vi "IR Stimulus DLL (SubVI).vi"(5 "GALVO Calibration Data":T1, 7 "Cycle Time (ms)":i32=50, 8 "LASER Intensity (%)":dbl format="%#_13g", 11 "irData":i32[](array[numeric])) -> (0 "Max. LASER Power (W)":dbl, 3 "daqData":dbl[][](array[numeric]))   [LabVIEW 2020]
uses:
  Controls (HOST)/IR GALVO Cal Data.ctl
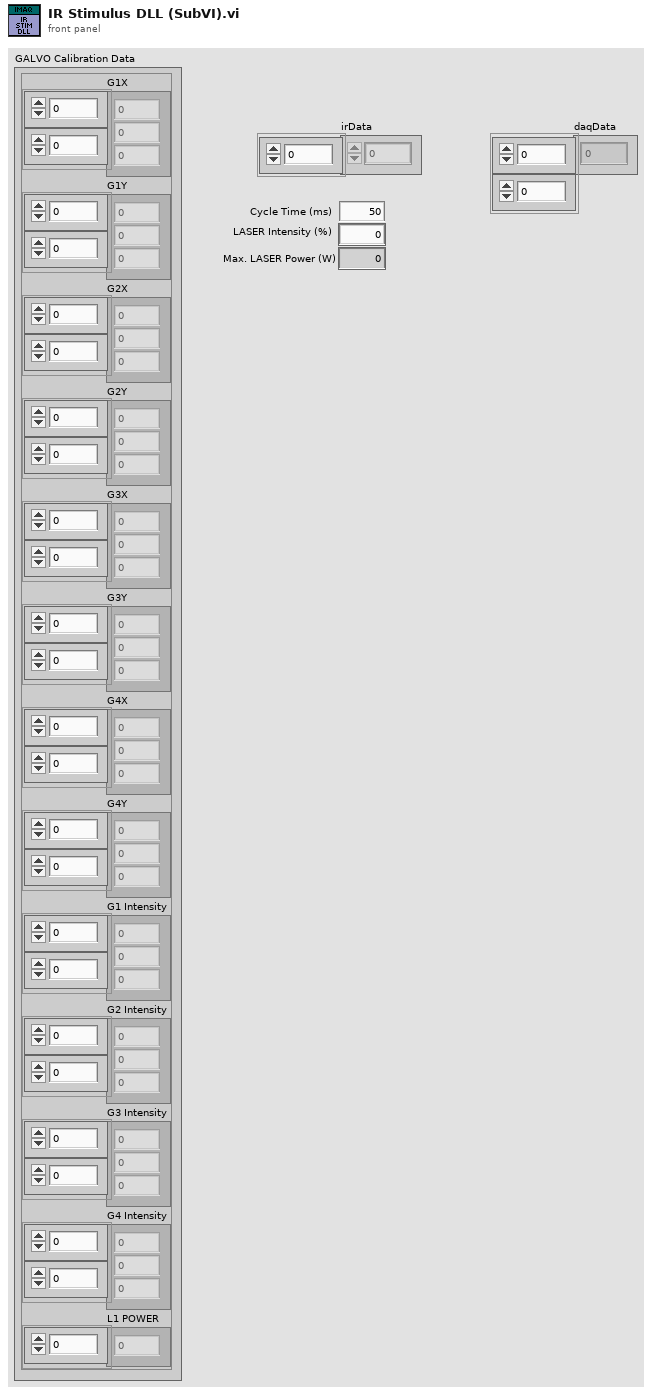
[diagram p1: front panel]
types:
  T1 = typedef "IR GALVO Cal Data.ctl" = cluster{"G1X":dbl[][], "G1Y":dbl[][], "G2X":dbl[][], "G2Y":dbl[][], "G3X":dbl[][], "G3Y":dbl[][], "G4X":dbl[][], "G4Y":dbl[][], "G1 Intensity":dbl[][], "G2 Intensity":dbl[][], "G3 Intensity":dbl[][], "G4 Intensity":dbl[][], "L1 POWER":dbl[]}
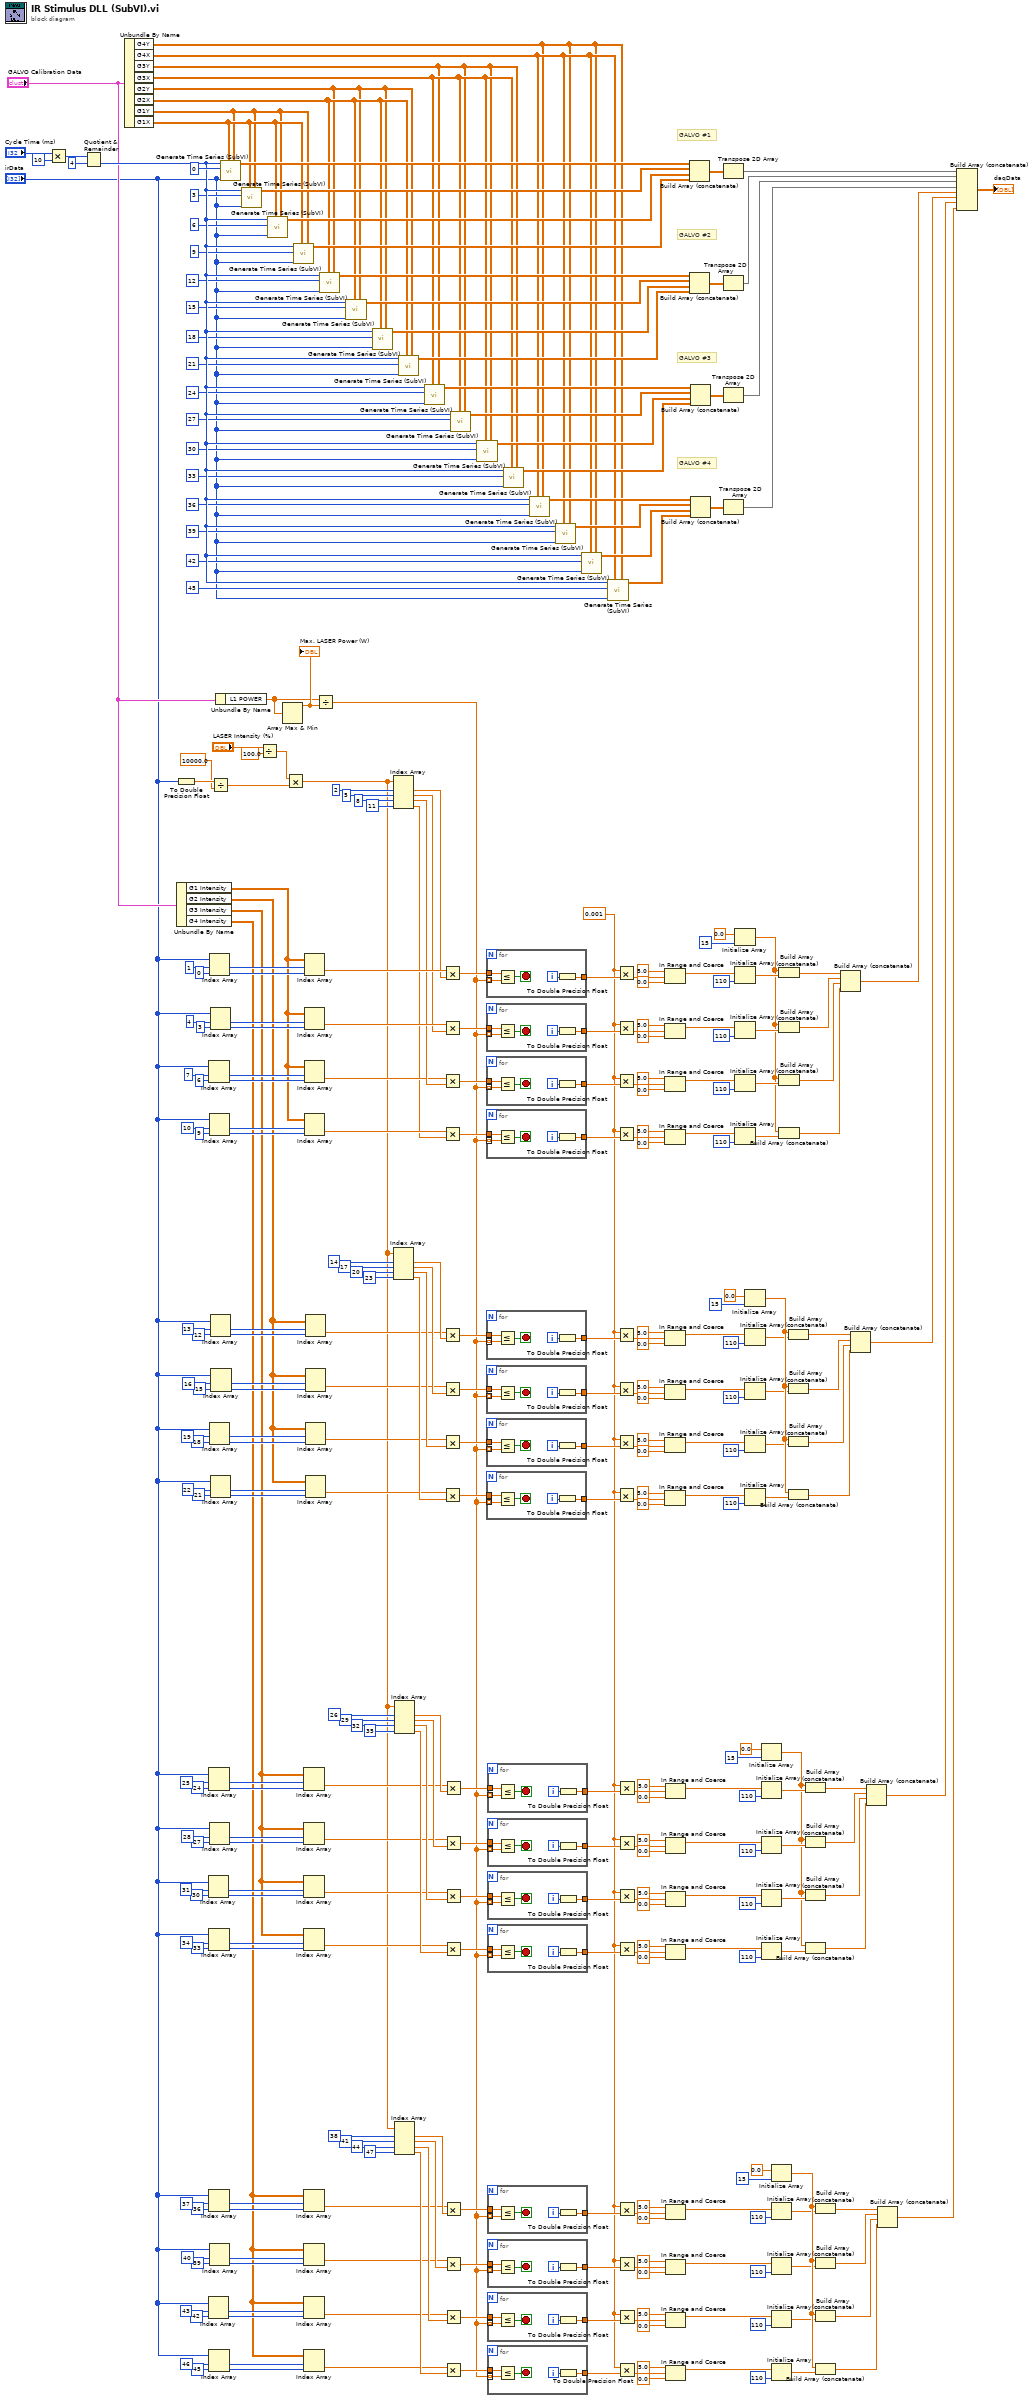
[diagram p0: block diagram]
diagram:
  w68 = 0.001 ("x")
  # "GALVO #4"
  # "GALVO #3"
  # "GALVO #2"
  # "GALVO #1"
  n1 = Multiply(x="Cycle Time (ms)", y=10) -> (x*y=w341:i32)
  n2 = Quotient & Remainder(x=w341, y=4) -> (floor(x/y)=w338:i32)  [unwired: 1 out]
  n3 = Unbundle By Name("GALVO Calibration Data") -> ("G4Y"=w290:dbl[][], "G4X"=w291:dbl[][], "G3Y"=w292:dbl[][], "G3X"=w293:dbl[][], "G2Y"=w294:dbl[][], "G2X"=w295:dbl[][], "G1Y"=w296:dbl[][], "G1X"=w297:dbl[][])
  n4 = To Double Precision Float(number="irData") -> (double precision float=w209:dbl[])
  n5 = Unbundle By Name("GALVO Calibration Data") -> ("G1 Intensity"=w256:dbl[][], "G2 Intensity"=w239:dbl[][], "G3 Intensity"=w238:dbl[][], "G4 Intensity"=w221:dbl[][])
  n6 = Index Array(array="irData", index #1=31 ("index"), index #2=30 ("index")) -> (element #1=w241:i32, element #2=w242:i32)
  n7 = Index Array(array="irData", index #1=43 ("index"), index #2=42 ("index")) -> (element #1=w236:i32, element #2=w235:i32)
  n8 = Index Array(array="irData", index #1=7 ("index"), index #2=6 ("index")) -> (element #1=w275:i32, element #2=w276:i32)
  n9 = Index Array(array="irData", index #1=25 ("index"), index #2=24 ("index")) -> (element #1=w254:i32, element #2=w253:i32)
  n10 = Index Array(array="irData", index #1=34 ("index"), index #2=33 ("index")) -> (element #1=w246:i32, element #2=w245:i32)
  n11 = Index Array(array="irData", index #1=37 ("index"), index #2=36 ("index")) -> (element #1=w223:i32, element #2=w224:i32)
  n12 = Index Array(array="irData", index #1=46 ("index"), index #2=45 ("index")) -> (element #1=w231:i32, element #2=w232:i32)
  n13 = Index Array(array="irData", index #1=1 ("index"), index #2=0 ("index")) -> (element #1=w288:i32, element #2=w287:i32)
  n14 = Index Array(array="irData", index #1=10 ("index"), index #2=9 ("index")) -> (element #1=w280:i32, element #2=w279:i32)
  n15 = Index Array(array="irData", index #1=19 ("index"), index #2=18 ("index")) -> (element #1=w271:i32, element #2=w270:i32)
  n16 = Index Array(array="irData", index #1=28 ("index"), index #2=27 ("index")) -> (element #1=w249:i32, element #2=w250:i32)
  n17 = Index Array(array="irData", index #1=40 ("index"), index #2=39 ("index")) -> (element #1=w228:i32, element #2=w227:i32)
  n18 = Index Array(array="irData", index #1=4 ("index"), index #2=3 ("index")) -> (element #1=w283:i32, element #2=w284:i32)
  n19 = Index Array(array="irData", index #1=13 ("index"), index #2=12 ("index")) -> (element #1=w258:i32, element #2=w259:i32)
  n20 = Index Array(array="irData", index #1=22 ("index"), index #2=21 ("index")) -> (element #1=w266:i32, element #2=w267:i32)
  n21 = Divide(x=w209, y=10000.0 ("LASER Intensity (%)")) -> (x/y=w208:dbl[])
  n22 = Index Array(array="irData", index #1=16 ("index"), index #2=15 ("index")) -> (element #1=w263:i32, element #2=w262:i32)
  n23 = Unbundle By Name("GALVO Calibration Data") -> ("L1 POWER"=w216:dbl[])
  n24 = call "Generate Time Series (SubVI).vi"("GY"=w296, "GX"=w297, "irData"="irData", "Start Index"=0, "N Steps"=w338) -> ("daqData"=w322:dbl[][])  [unwired: 6 in]
  n25 = call "Generate Time Series (SubVI).vi"("GY"=w296, "GX"=w297, "irData"="irData", "Start Index"=3, "N Steps"=w338) -> ("daqData"=w321:dbl[][])  [unwired: 6 in]
  n26 = Divide(x="LASER Intensity (%)", y=100.0 ("x")) -> (x/y=w86:dbl)
  n27 = call "Generate Time Series (SubVI).vi"("GY"=w296, "GX"=w297, "irData"="irData", "Start Index"=6, "N Steps"=w338) -> ("daqData"=w320:dbl[][])  [unwired: 6 in]
  n28 = Array Max & Min(array=w216) -> (max value=w217:dbl)  [unwired: 3 out]
  "Max. LASER Power (W)" <- w217
  n29 = Multiply(x=w86, y=w208) -> (x*y=w92:dbl[])
  n30 = call "Generate Time Series (SubVI).vi"("GY"=w296, "GX"=w297, "irData"="irData", "Start Index"=9, "N Steps"=w338) -> ("daqData"=w319:dbl[][])  [unwired: 6 in]
  n31 = Index Array(array=w238, index (row)=w254, index (col)=w253) -> (element=w120:dbl)
  n32 = Index Array(array=w238, index (row)=w249, index (col)=w250) -> (element=w119:dbl)
  n33 = Index Array(array=w238, index (row)=w241, index (col)=w242) -> (element=w118:dbl)
  n34 = Index Array(array=w238, index (row)=w246, index (col)=w245) -> (element=w117:dbl)
  n35 = Index Array(array=w221, index (row)=w223, index (col)=w224) -> (element=w90:dbl)
  n36 = Index Array(array=w221, index (row)=w228, index (col)=w227) -> (element=w89:dbl)
  n37 = Index Array(array=w221, index (row)=w236, index (col)=w235) -> (element=w88:dbl)
  n38 = Index Array(array=w221, index (row)=w231, index (col)=w232) -> (element=w87:dbl)
  n39 = Index Array(array=w256, index (row)=w288, index (col)=w287) -> (element=w201:dbl)
  n40 = Index Array(array=w256, index (row)=w283, index (col)=w284) -> (element=w194:dbl)
  n41 = Index Array(array=w256, index (row)=w275, index (col)=w276) -> (element=w183:dbl)
  n42 = Index Array(array=w256, index (row)=w280, index (col)=w279) -> (element=w176:dbl)
  n43 = Index Array(array=w239, index (row)=w258, index (col)=w259) -> (element=w148:dbl)
  n44 = Index Array(array=w239, index (row)=w263, index (col)=w262) -> (element=w147:dbl)
  n45 = Index Array(array=w239, index (row)=w271, index (col)=w270) -> (element=w146:dbl)
  n46 = Index Array(array=w239, index (row)=w266, index (col)=w267) -> (element=w145:dbl)
  n47 = Divide(x=w216, y=w217) -> (x/y=w91:dbl[])
  n48 = call "Generate Time Series (SubVI).vi"("GY"=w294, "GX"=w295, "irData"="irData", "Start Index"=12, "N Steps"=w338) -> ("daqData"=w318:dbl[][])  [unwired: 6 in]
  n49 = call "Generate Time Series (SubVI).vi"("GY"=w294, "GX"=w295, "irData"="irData", "Start Index"=15, "N Steps"=w338) -> ("daqData"=w317:dbl[][])  [unwired: 6 in]
  n50 = call "Generate Time Series (SubVI).vi"("GY"=w294, "GX"=w295, "irData"="irData", "Start Index"=18, "N Steps"=w338) -> ("daqData"=w316:dbl[][])  [unwired: 6 in]
  n51 = Index Array(array=w92, index #1=2 ("index"), index #2=5 ("index"), index #3=8 ("index"), index #4=11 ("index")) -> (element #1=w193:dbl, element #2=w185:dbl, element #3=w184:dbl, element #4=w175:dbl)
  n52 = Index Array(array=w92, index #1=14 ("index"), index #2=17 ("index"), index #3=20 ("index"), index #4=23 ("index")) -> (element #1=w161:dbl, element #2=w166:dbl, element #3=w167:dbl, element #4=w172:dbl)
  n53 = Index Array(array=w92, index #1=26 ("index"), index #2=29 ("index"), index #3=32 ("index"), index #4=35 ("index")) -> (element #1=w132:dbl, element #2=w127:dbl, element #3=w126:dbl, element #4=w121:dbl)
  n54 = Index Array(array=w92, index #1=38 ("index"), index #2=41 ("index"), index #3=44 ("index"), index #4=47 ("index")) -> (element #1=w105:dbl, element #2=w110:dbl, element #3=w111:dbl, element #4=w116:dbl)
  n55 = call "Generate Time Series (SubVI).vi"("GY"=w294, "GX"=w295, "irData"="irData", "Start Index"=21, "N Steps"=w338) -> ("daqData"=w315:dbl[][])  [unwired: 6 in]
  n56 = call "Generate Time Series (SubVI).vi"("GY"=w292, "GX"=w293, "irData"="irData", "Start Index"=24, "N Steps"=w338) -> ("daqData"=w314:dbl[][])  [unwired: 6 in]
  n57 = Multiply(x=w201, y=w193) -> (x*y=w202:dbl)
  n58 = Multiply(x=w194, y=w185) -> (x*y=w200:dbl)
  n59 = Multiply(x=w183, y=w184) -> (x*y=w186:dbl)
  n60 = Multiply(x=w176, y=w175) -> (x*y=w182:dbl)
  n61 = Multiply(x=w148, y=w161) -> (x*y=w156:dbl)
  n62 = Multiply(x=w147, y=w166) -> (x*y=w157:dbl)
  n63 = Multiply(x=w146, y=w167) -> (x*y=w165:dbl)
  n64 = Multiply(x=w145, y=w172) -> (x*y=w168:dbl)
  n65 = Multiply(x=w120, y=w132) -> (x*y=w137:dbl)
  n66 = Multiply(x=w119, y=w127) -> (x*y=w136:dbl)
  n67 = Multiply(x=w118, y=w126) -> (x*y=w128:dbl)
  n68 = Multiply(x=w117, y=w121) -> (x*y=w125:dbl)
  n69 = Multiply(x=w90, y=w105) -> (x*y=w100:dbl)
  n70 = Multiply(x=w89, y=w110) -> (x*y=w101:dbl)
  n71 = Multiply(x=w88, y=w111) -> (x*y=w109:dbl)
  n72 = Multiply(x=w87, y=w116) -> (x*y=w112:dbl)
  n73 = call "Generate Time Series (SubVI).vi"("GY"=w292, "GX"=w293, "irData"="irData", "Start Index"=27, "N Steps"=w338) -> ("daqData"=w313:dbl[][])  [unwired: 6 in]
  n74 = call "Generate Time Series (SubVI).vi"("GY"=w292, "GX"=w293, "irData"="irData", "Start Index"=30, "N Steps"=w338) -> ("daqData"=w312:dbl[][])  [unwired: 6 in]
  n75 = for {
    tunnel: w91 -> [w348] mode=indexing
    tunnel: [w345] -> w215
    tunnel: w202 -> [w344]
    i -> [w346]
    stop <- w347 stop-if-true
    n76 = Less Or Equal?(x=w344, y=w348) -> (x <= y?=w347:bool)
    n77 = To Double Precision Float(number=w346) -> (double precision float=w345:dbl)
  }
  n78 = for {
    tunnel: w91 -> [w353] mode=indexing
    tunnel: [w350] -> w197
    tunnel: w200 -> [w349]
    i -> [w351]
    stop <- w352 stop-if-true
    n79 = Less Or Equal?(x=w349, y=w353) -> (x <= y?=w352:bool)
    n80 = To Double Precision Float(number=w351) -> (double precision float=w350:dbl)
  }
  n81 = for {
    tunnel: w91 -> [w358] mode=indexing
    tunnel: [w355] -> w189
    tunnel: w186 -> [w354]
    i -> [w356]
    stop <- w357 stop-if-true
    n82 = Less Or Equal?(x=w354, y=w358) -> (x <= y?=w357:bool)
    n83 = To Double Precision Float(number=w356) -> (double precision float=w355:dbl)
  }
  n84 = for {
    tunnel: w91 -> [w363] mode=indexing
    tunnel: [w360] -> w179
    tunnel: w182 -> [w359]
    i -> [w361]
    stop <- w362 stop-if-true
    n85 = Less Or Equal?(x=w359, y=w363) -> (x <= y?=w362:bool)
    n86 = To Double Precision Float(number=w361) -> (double precision float=w360:dbl)
  }
  n87 = for {
    tunnel: w91 -> [w368] mode=indexing
    tunnel: [w365] -> w151
    tunnel: w156 -> [w364]
    i -> [w366]
    stop <- w367 stop-if-true
    n88 = Less Or Equal?(x=w364, y=w368) -> (x <= y?=w367:bool)
    n89 = To Double Precision Float(number=w366) -> (double precision float=w365:dbl)
  }
  n90 = for {
    tunnel: w91 -> [w373] mode=indexing
    tunnel: [w370] -> w158
    tunnel: w157 -> [w369]
    i -> [w371]
    stop <- w372 stop-if-true
    n91 = Less Or Equal?(x=w369, y=w373) -> (x <= y?=w372:bool)
    n92 = To Double Precision Float(number=w371) -> (double precision float=w370:dbl)
  }
  n93 = for {
    tunnel: w91 -> [w378] mode=indexing
    tunnel: [w375] -> w164
    tunnel: w165 -> [w374]
    i -> [w376]
    stop <- w377 stop-if-true
    n94 = Less Or Equal?(x=w374, y=w378) -> (x <= y?=w377:bool)
    n95 = To Double Precision Float(number=w376) -> (double precision float=w375:dbl)
  }
  n96 = for {
    tunnel: w91 -> [w383] mode=indexing
    tunnel: [w380] -> w169
    tunnel: w168 -> [w379]
    i -> [w381]
    stop <- w382 stop-if-true
    n97 = Less Or Equal?(x=w379, y=w383) -> (x <= y?=w382:bool)
    n98 = To Double Precision Float(number=w381) -> (double precision float=w380:dbl)
  }
  n99 = for {
    tunnel: w91 -> [w388] mode=indexing
    tunnel: [w385] -> w142
    tunnel: w137 -> [w384]
    i -> [w386]
    stop <- w387 stop-if-true
    n100 = Less Or Equal?(x=w384, y=w388) -> (x <= y?=w387:bool)
    n101 = To Double Precision Float(number=w386) -> (double precision float=w385:dbl)
  }
  n102 = for {
    tunnel: w91 -> [w393] mode=indexing
    tunnel: [w390] -> w135
    tunnel: w136 -> [w389]
    i -> [w391]
    stop <- w392 stop-if-true
    n103 = Less Or Equal?(x=w389, y=w393) -> (x <= y?=w392:bool)
    n104 = To Double Precision Float(number=w391) -> (double precision float=w390:dbl)
  }
  n105 = for {
    tunnel: w91 -> [w398] mode=indexing
    tunnel: [w395] -> w129
    tunnel: w128 -> [w394]
    i -> [w396]
    stop <- w397 stop-if-true
    n106 = Less Or Equal?(x=w394, y=w398) -> (x <= y?=w397:bool)
    n107 = To Double Precision Float(number=w396) -> (double precision float=w395:dbl)
  }
  n108 = for {
    tunnel: w91 -> [w403] mode=indexing
    tunnel: [w400] -> w124
    tunnel: w125 -> [w399]
    i -> [w401]
    stop <- w402 stop-if-true
    n109 = Less Or Equal?(x=w399, y=w403) -> (x <= y?=w402:bool)
    n110 = To Double Precision Float(number=w401) -> (double precision float=w400:dbl)
  }
  n111 = for {
    tunnel: w91 -> [w408] mode=indexing
    tunnel: [w405] -> w95
    tunnel: w100 -> [w404]
    i -> [w406]
    stop <- w407 stop-if-true
    n112 = Less Or Equal?(x=w404, y=w408) -> (x <= y?=w407:bool)
    n113 = To Double Precision Float(number=w406) -> (double precision float=w405:dbl)
  }
  n114 = for {
    tunnel: w91 -> [w413] mode=indexing
    tunnel: [w410] -> w102
    tunnel: w101 -> [w409]
    i -> [w411]
    stop <- w412 stop-if-true
    n115 = Less Or Equal?(x=w409, y=w413) -> (x <= y?=w412:bool)
    n116 = To Double Precision Float(number=w411) -> (double precision float=w410:dbl)
  }
  n117 = for {
    tunnel: w91 -> [w418] mode=indexing
    tunnel: [w415] -> w108
    tunnel: w109 -> [w414]
    i -> [w416]
    stop <- w417 stop-if-true
    n118 = Less Or Equal?(x=w414, y=w418) -> (x <= y?=w417:bool)
    n119 = To Double Precision Float(number=w416) -> (double precision float=w415:dbl)
  }
  n120 = for {
    tunnel: w91 -> [w423] mode=indexing
    tunnel: [w420] -> w113
    tunnel: w112 -> [w419]
    i -> [w421]
    stop <- w422 stop-if-true
    n121 = Less Or Equal?(x=w419, y=w423) -> (x <= y?=w422:bool)
    n122 = To Double Precision Float(number=w421) -> (double precision float=w420:dbl)
  }
  n123 = call "Generate Time Series (SubVI).vi"("GY"=w292, "GX"=w293, "irData"="irData", "Start Index"=33, "N Steps"=w338) -> ("daqData"=w311:dbl[][])  [unwired: 6 in]
  n124 = call "Generate Time Series (SubVI).vi"("GY"=w290, "GX"=w291, "irData"="irData", "Start Index"=36, "N Steps"=w338) -> ("daqData"=w310:dbl[][])  [unwired: 6 in]
  n125 = call "Generate Time Series (SubVI).vi"("GY"=w290, "GX"=w291, "irData"="irData", "Start Index"=39, "N Steps"=w338) -> ("daqData"=w309:dbl[][])  [unwired: 6 in]
  n126 = call "Generate Time Series (SubVI).vi"("GY"=w290, "GX"=w291, "irData"="irData", "Start Index"=42, "N Steps"=w338) -> ("daqData"=w308:dbl[][])  [unwired: 6 in]
  n127 = call "Generate Time Series (SubVI).vi"("GY"=w290, "GX"=w291, "irData"="irData", "Start Index"=45, "N Steps"=w338) -> ("daqData"=w307:dbl[][])  [unwired: 6 in]
  n128 = Multiply(x=w68, y=w215) -> (x*y=w84:dbl)
  n129 = Multiply(x=w68, y=w197) -> (x*y=w83:dbl)
  n130 = Multiply(x=w68, y=w189) -> (x*y=w82:dbl)
  n131 = Multiply(x=w68, y=w179) -> (x*y=w81:dbl)
  n132 = Multiply(x=w68, y=w151) -> (x*y=w80:dbl)
  n133 = Multiply(x=w68, y=w158) -> (x*y=w79:dbl)
  n134 = Multiply(x=w68, y=w164) -> (x*y=w78:dbl)
  n135 = Multiply(x=w68, y=w169) -> (x*y=w77:dbl)
  n136 = Multiply(x=w68, y=w142) -> (x*y=w76:dbl)
  n137 = Multiply(x=w68, y=w135) -> (x*y=w75:dbl)
  n138 = Multiply(x=w68, y=w129) -> (x*y=w74:dbl)
  n139 = Multiply(x=w68, y=w124) -> (x*y=w73:dbl)
  n140 = Multiply(x=w68, y=w95) -> (x*y=w72:dbl)
  n141 = Multiply(x=w68, y=w102) -> (x*y=w71:dbl)
  n142 = Multiply(x=w68, y=w108) -> (x*y=w70:dbl)
  n143 = Multiply(x=w68, y=w113) -> (x*y=w69:dbl)
  n144 = In Range and Coerce(upper limit=5.0, x=w84, lower limit=0.0) -> (coerced(x)=w205:dbl)  [unwired: 1 out]
  n145 = In Range and Coerce(upper limit=5.0, x=w83, lower limit=0.0) -> (coerced(x)=w198:dbl)  [unwired: 1 out]
  n146 = In Range and Coerce(upper limit=5.0, x=w82, lower limit=0.0) -> (coerced(x)=w188:dbl)  [unwired: 1 out]
  n147 = In Range and Coerce(upper limit=5.0, x=w81, lower limit=0.0) -> (coerced(x)=w180:dbl)  [unwired: 1 out]
  n148 = In Range and Coerce(upper limit=5.0, x=w80, lower limit=0.0) -> (coerced(x)=w45:dbl)  [unwired: 1 out]
  n149 = In Range and Coerce(upper limit=5.0, x=w79, lower limit=0.0) -> (coerced(x)=w44:dbl)  [unwired: 1 out]
  n150 = In Range and Coerce(upper limit=5.0, x=w78, lower limit=0.0) -> (coerced(x)=w43:dbl)  [unwired: 1 out]
  n151 = In Range and Coerce(upper limit=5.0, x=w77, lower limit=0.0) -> (coerced(x)=w42:dbl)  [unwired: 1 out]
  n152 = In Range and Coerce(upper limit=5.0, x=w76, lower limit=0.0) -> (coerced(x)=w25:dbl)  [unwired: 1 out]
  n153 = In Range and Coerce(upper limit=5.0, x=w75, lower limit=0.0) -> (coerced(x)=w24:dbl)  [unwired: 1 out]
  n154 = In Range and Coerce(upper limit=5.0, x=w74, lower limit=0.0) -> (coerced(x)=w23:dbl)  [unwired: 1 out]
  n155 = In Range and Coerce(upper limit=5.0, x=w73, lower limit=0.0) -> (coerced(x)=w22:dbl)  [unwired: 1 out]
  n156 = In Range and Coerce(upper limit=5.0, x=w72, lower limit=0.0) -> (coerced(x)=w5:dbl)  [unwired: 1 out]
  n157 = In Range and Coerce(upper limit=5.0, x=w71, lower limit=0.0) -> (coerced(x)=w4:dbl)  [unwired: 1 out]
  n158 = In Range and Coerce(upper limit=5.0, x=w70, lower limit=0.0) -> (coerced(x)=w3:dbl)  [unwired: 1 out]
  n159 = In Range and Coerce(upper limit=5.0, x=w69, lower limit=0.0) -> (coerced(x)=w2:dbl)  [unwired: 1 out]
  n160 = Build Array (concatenate)(w322, w321, w320, w319) -> (w306:dbl[][])
  n161 = Build Array (concatenate)(w318, w317, w316, w315) -> (w305:dbl[][])
  n162 = Build Array (concatenate)(w314, w313, w312, w311) -> (w304:dbl[][])
  n163 = Build Array (concatenate)(w310, w309, w308, w307) -> (w303:dbl[][])
  n164 = Transpose 2D Array(2D array=w306) -> (transposed array=w301:dbl[][])
  n165 = Transpose 2D Array(2D array=w305) -> (transposed array=w300:dbl[][])
  n166 = Transpose 2D Array(2D array=w304) -> (transposed array=w299:dbl[][])
  n167 = Transpose 2D Array(2D array=w303) -> (transposed array=w298:dbl[][])
  n168 = Initialize Array(0.0 ("lower limit"), 15 ("dimension size")) -> (w61:dbl[])
  n169 = Initialize Array(w205, 110 ("dimension size")) -> (w203:dbl[])
  n170 = Initialize Array(w198, 110 ("dimension size")) -> (w192:dbl[])
  n171 = Initialize Array(w188, 110 ("dimension size")) -> (w174:dbl[])
  n172 = Initialize Array(w180, 110 ("dimension size")) -> (w173:dbl[])
  n173 = Initialize Array(0.0 ("lower limit"), 15 ("dimension size")) -> (w60:dbl[])
  n174 = Initialize Array(w45, 110 ("dimension size")) -> (w47:dbl[])
  n175 = Initialize Array(w44, 110 ("dimension size")) -> (w49:dbl[])
  n176 = Initialize Array(w43, 110 ("dimension size")) -> (w52:dbl[])
  n177 = Initialize Array(w42, 110 ("dimension size")) -> (w53:dbl[])
  n178 = Initialize Array(0.0 ("lower limit"), 15 ("dimension size")) -> (w26:dbl[])
  n179 = Initialize Array(w25, 110 ("dimension size")) -> (w39:dbl[])
  n180 = Initialize Array(w24, 110 ("dimension size")) -> (w37:dbl[])
  n181 = Initialize Array(w23, 110 ("dimension size")) -> (w34:dbl[])
  n182 = Initialize Array(w22, 110 ("dimension size")) -> (w33:dbl[])
  n183 = Initialize Array(0.0 ("lower limit"), 15 ("dimension size")) -> (w20:dbl[])
  n184 = Initialize Array(w5, 110 ("dimension size")) -> (w7:dbl[])
  n185 = Initialize Array(w4, 110 ("dimension size")) -> (w9:dbl[])
  n186 = Initialize Array(w3, 110 ("dimension size")) -> (w12:dbl[])
  n187 = Initialize Array(w2, 110 ("dimension size")) -> (w13:dbl[])
  n188 = Build Array (concatenate)(w61, w203) -> (w65:dbl[])
  n189 = Build Array (concatenate)(w61, w192) -> (w64:dbl[])
  n190 = Build Array (concatenate)(w61, w174) -> (w63:dbl[])
  n191 = Build Array (concatenate)(w61, w173) -> (w62:dbl[])
  n192 = Build Array (concatenate)(w60, w47) -> (w56:dbl[])
  n193 = Build Array (concatenate)(w60, w49) -> (w57:dbl[])
  n194 = Build Array (concatenate)(w60, w52) -> (w58:dbl[])
  n195 = Build Array (concatenate)(w60, w53) -> (w59:dbl[])
  n196 = Build Array (concatenate)(w26, w39) -> (w30:dbl[])
  n197 = Build Array (concatenate)(w26, w37) -> (w29:dbl[])
  n198 = Build Array (concatenate)(w26, w34) -> (w28:dbl[])
  n199 = Build Array (concatenate)(w26, w33) -> (w27:dbl[])
  n200 = Build Array (concatenate)(w20, w7) -> (w16:dbl[])
  n201 = Build Array (concatenate)(w20, w9) -> (w17:dbl[])
  n202 = Build Array (concatenate)(w20, w12) -> (w18:dbl[])
  n203 = Build Array (concatenate)(w20, w13) -> (w19:dbl[])
  n204 = Build Array (concatenate)(w65, w64, w63, w62) -> (w273:dbl[])
  n205 = Build Array (concatenate)(w56, w57, w58, w59) -> (w41:dbl[])
  n206 = Build Array (concatenate)(w30, w29, w28, w27) -> (w21:dbl[])
  n207 = Build Array (concatenate)(w16, w17, w18, w19) -> (w1:dbl[])
  n208 = Build Array (concatenate)(w301, w300, w299, w298, w273, w41, w21, w1) -> (→"daqData":dbl[][])
